vi "calibration_and_perspective.vi"() -> ()   [LabVIEW 2011]
panel:
  in  "error in":errorcluster
  out "Image Out 2":T1(plugin-control)
  out "Image Out":T1(plugin-control)
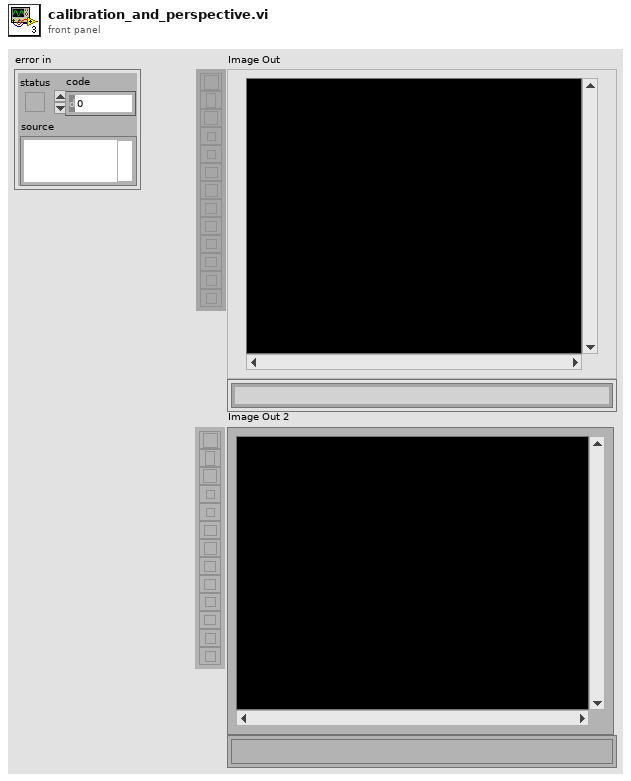
[diagram p1: front panel]
types:
  T1 = typedef "IMAQ Image.ctl" = refnum<image>
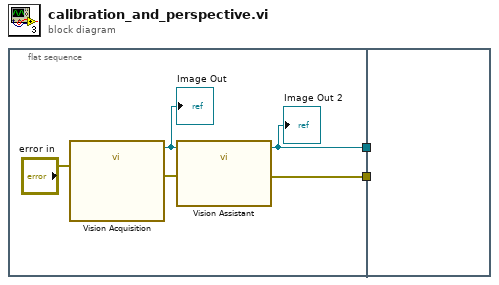
[diagram p0: block diagram]
diagram:
  n1 = flat-sequence {
    tunnel: [w5] -> w2
    tunnel: [w4] -> w1
    tunnel: w2 -> [_]
    tunnel: w1 -> [_]
    frame #0 {
      n2 = call "Vision Acquisition"("error in"="error in") -> ("Image Out"=w3:T1, "error out"=w7:errorcluster)  [unwired: 25 in]
      "Image Out" <- w3
      n3 = call "Vision Assistant"("Image In"=w3, "error in"=w7) -> ("Image Out"=w4:T1, "error out"=w5:errorcluster)  [unwired: 24 in]
      "Image Out 2" <- w4
    }
    frame #1 {
    }
  }
